vi "MICSD Get Register.vi"(7 "Execute on Remote?(F)":bool, 8 "error in (no error)":errorcluster, 10 "Address":u16 format="%04x", 11 "VISA Resource Name":refnum<visa-resource-name>) -> (0 "error out":errorcluster, 2 "Data":u8 format="%02x", 3 "dup VISA Resource Name":refnum<visa-resource-name>)   [LabVIEW 2010]
uses:
  <vilib>/Instr/_visa.llb/VISA Configure Serial Port (Instr).vi
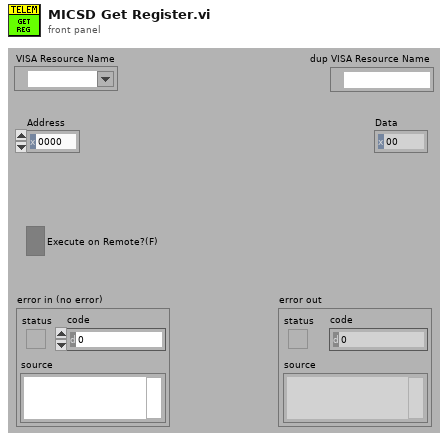
[diagram p1: front panel]
types:
  T1 = cluster{"Command Token":u8, "Length":u16, "Pack Data":u8[]}
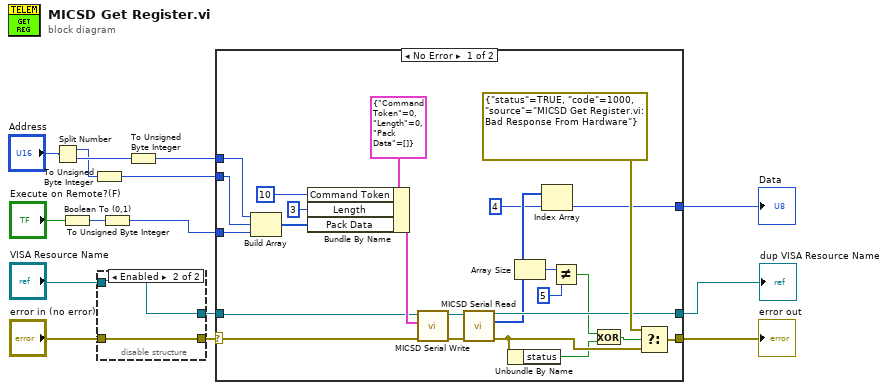
[diagram p0: block diagram]
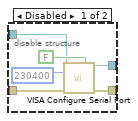
[diagram p2: hidden frame]
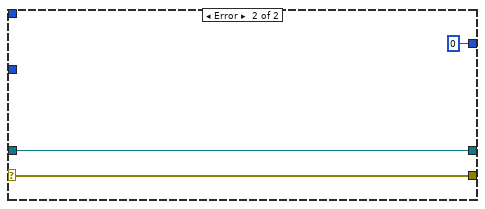
[diagram p3: hidden frame]
diagram:
  n1 = Split Number(x="Address") -> (hi(x)=w8:u8, lo(x)=w9:u8)
  n2 = Boolean To (0,1)(Boolean="Execute on Remote?(F)") -> (0, 1=w6:i16)
  n3 = To Unsigned Byte Integer(number=w8) -> (unsigned 8bit integer=w2:u8)
  n4 = disable-structure shown="Enabled" {
    disable-tunnel: [w19 w22] -> w14
    disable-tunnel: "error in (no error)" -> [w18 w22]
    disable-tunnel: "VISA Resource Name" -> [w17 w23]
    disable-tunnel: [w16 w23] -> w11
    frame Disabled {
      n5 = call-poly "VISA Configure Serial Port"("VISA resource name"=w17, "Enable Termination\nChar (T)"=FALSE ("Enable Termination\nChar (T)"), "baud rate (9600)"=u32 230400, "error in (no error)"=w18) -> ("VISA resource name out"=w16:refnum<visa-resource-name>, "error out"=w19:errorcluster)  [unwired: 10 in]
    }
    frame Enabled {
    }
  }
  n6 = To Unsigned Byte Integer(number=w6) -> (unsigned 8bit integer=w1:u8)
  n7 = To Unsigned Byte Integer(number=w9) -> (unsigned 8bit integer=w3:u8)
  n8 = case shown="No Error" w14 {
    selector: w14 -> [w45 w50]
    tunnel: [w35 w50] -> w10
    tunnel: w11 -> [w44 w49]
    tunnel: [w36 w49] -> w15
    tunnel: [w32 u8 0 ("Source")] -> w4
    tunnel: w3 -> [w27 _]
    tunnel: w2 -> [w24 _]
    tunnel: w1 -> [w25 _]
    frame No Error {
      n9 = Build Array(w27, w24, w25) -> (w26:u8[])
      n10 = Bundle By Name(cluster=T1 {"Command Token"=0, "Length"=0, "Pack Data"=[]} ("Write Data"), "Command Token"=u16 10 ("Length"), "Length"=u16 3, "Pack Data"=w26) -> (w47:T1)
      n11 = call "MICSD Serial Write.vi"("error in (no error)"=w45, "Write Data"=w47, "VISA Resource Name"=w44) -> ("error out"=w41:errorcluster, "DUP Visa Resource Name"=w42:refnum<visa-resource-name>)  [unwired: 7 in]
      n12 = call "MICSD Serial Read.vi"("error in (no error)"=w41, "VISA Resource Name"=w42) -> ("error out"=w31:errorcluster, "Read Data"=w34:u8[], "DUP Visa Resource Name"=w36:refnum<visa-resource-name>)  [unwired: 7 in]
      n13 = Unbundle By Name(w31) -> ("status"=w28:bool)
      n14 = Array Size(array=w34) -> (size(s)=w38:i32)
      n15 = Index Array(array=w34, index=4) -> (element=w32:u8)
      n16 = Not Equal?(x=w38, y=5) -> (x != y?=w29:bool)
      n17 = Exclusive Or(1:w28, 2:w29) -> (0:w30:bool)
      n18 = Select(t=errorcluster {"status"=TRUE, "code"=1000, "source"="MICSD Get Register.vi:  Bad Response From Hardware"} ("error IO"), s=w30, f=w31) -> (s? t:f=w35:errorcluster)
    }
    frame Error {
    }
  }
  "dup VISA Resource Name" <- w15
  "error out" <- w10
  "Data" <- w4
